vi "Event-Settings-source.vi"(7 "Settings source":T1, 8 "error in (no error)":errorcluster, 10 "Data ref. in":refnum<data-value>, 11 "UI ref. in":refnum<data-value>) -> (0 "error out":errorcluster, 2 "Data ref.":refnum<data-value>, 3 "UI ref.":refnum<data-value>)   [LabVIEW 2013, in "CameraVision.lvlib" / "CV-UI.lvclass"]
uses:
  CV-UI.lvclass
  Main/CV-Main.lvclass
  Settings-source.ctl
  Control-names.ctl
  CV-UI.lvclass/CV-UI.ctl
  Read Settings-source.vi
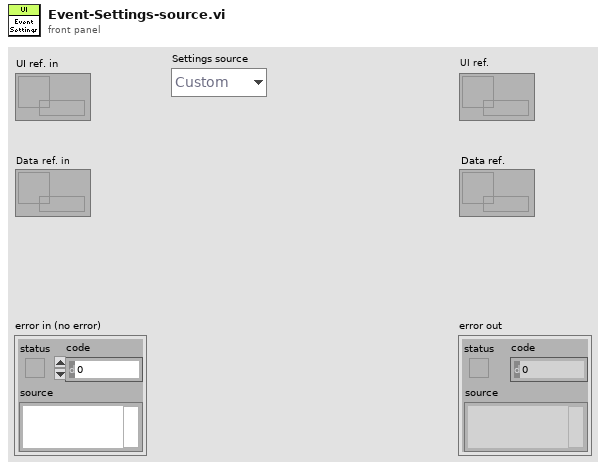
[diagram p1: front panel]
types:
  T1 = typedef "CameraVision.lvlib/CV-UI.lvclass/Settings-source.ctl" = enum16{"Custom", "Default", "Last used", "File"}
  T2 = typedef "CameraVision.lvlib/CV-UI.lvclass/Control-names.ctl" = enum16{"Start acquisition", "Activate", "Stop acquisition", "Settings type", "Load settings", "Save settings", "Import images", "Camera selector", "Image type selector", "Batch browser", "Image refresh", "Parameter tabs", "Displays", "Processing tabs", "Processing selector", "Map characteristic", "Show info", "Manual trigger"}
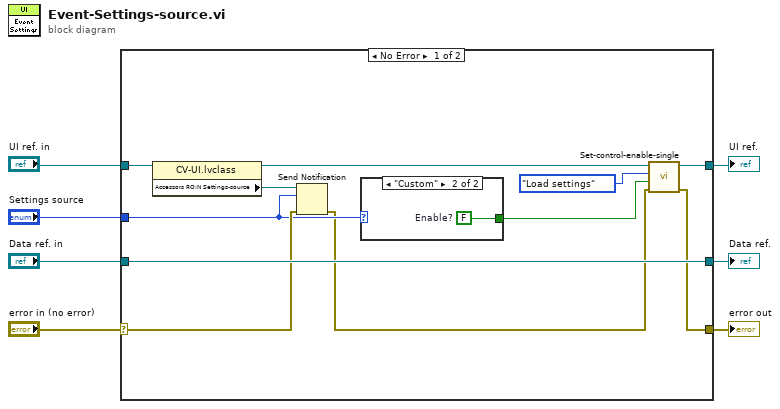
[diagram p0: block diagram]
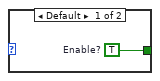
[diagram p2: hidden frame]
diagram:
  n1 = case shown="No Error" "error in (no error)" {
    selector: "error in (no error)" -> [w15 w23]
    tunnel: [w8 w23] -> w6
    tunnel: [w12 w22] -> w4
    tunnel: "UI ref. in" -> [w17 w22]
    tunnel: "Data ref. in" -> [w18 w21]
    tunnel: "Settings source" -> [w13 _]
    tunnel: [w18 w21] -> w2
    frame No Error {
      n2 = property class="CV-UI.lvclass"(reference=w17) -> (reference out=w14:refnum<data-value>, "Accessors RO:N Settings-source"=w16:refnum<notifier>)  [unwired: 1 in, 1 out]
      n3 = Send Notification(notification=w13, notifier=w16, error in (no error)=w15) -> (error out=w9:errorcluster)  [unwired: 1 out]
      n4 = case shown="\"Custom\"" w13 {
        tunnel: [w19 w20] -> w10
        frame Default {
          w19 = TRUE  # Enable?
        }
        frame "Custom" {
          w20 = FALSE  # Enable?
        }
      }
      n5 = call "Set-control-enable-single.vi"("error in (no error)"=w9, "Enable?"=w10, "Control name"=Control-names."Load settings", "UI ref. in"=w14) -> ("error out"=w8:errorcluster, "UI ref."=w12:refnum<data-value>)  [unwired: 6 in]
    }
    frame Error {
    }
  }
  "error out" <- w6
  "Data ref." <- w2
  "UI ref." <- w4
